vi "ZK组合命令区.vi"(7 "是否启用通讯通知":bool, 8 "error in (no error)":errorcluster, 9 "加标体积":sgl, 10 "组合命令区":T2, 11 "Slave ID":T1) -> (0 "error out":errorcluster)   [LabVIEW 2016, in "质控单元V2.lvlib"]
uses:
  <vilib>/Plasmionique/MB Master/MB_Master/MB_Master.lvclass
  <vilib>/Plasmionique/MB Master/MB Master.lvlib
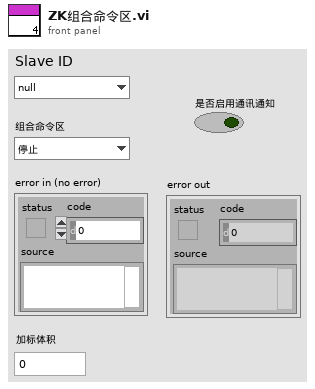
[diagram p1: front panel]
types:
  T1 = typedef "质控单元V2.lvlib/质控slave id.ctl" = enum16{"null", "氨氮", "总磷", "总氮", "CODMn", "CODCr"}
  T2 = typedef "质控单元V2.lvlib/质控组合命令区.ctl" = enum16{"停止", "进水样", "排废液", "进空气（搅拌）", "定量（反转定量）", "加标"}
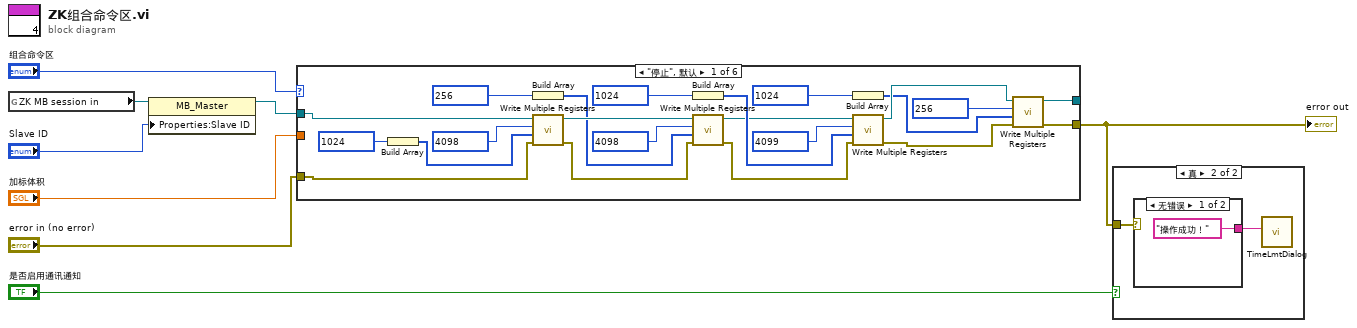
[diagram p0: block diagram]
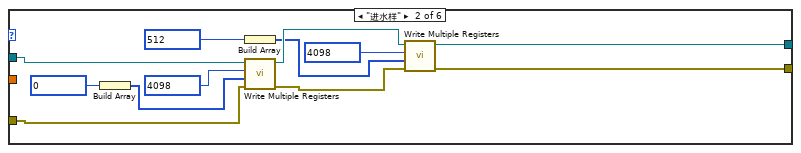
[diagram p2: hidden frame]
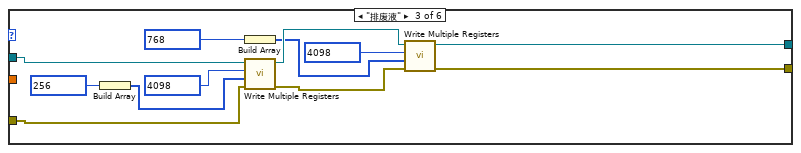
[diagram p3: hidden frame]
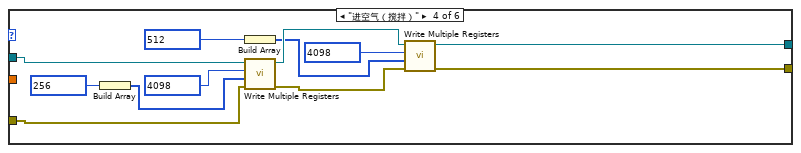
[diagram p4: hidden frame]
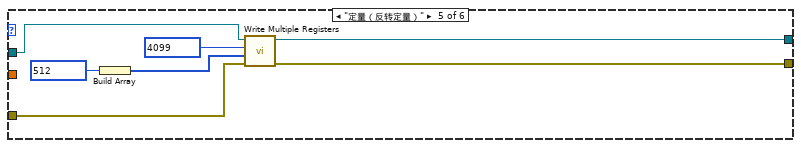
[diagram p5: hidden frame]
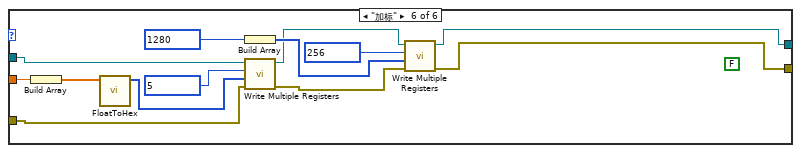
[diagram p6: hidden frame]
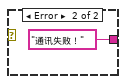
[diagram p8: hidden frame]
diagram:
  n1 = global read "ZK非断电保存全局变量.vi" "ZK MB session in"() -> (w8:refnum<class "MB_Master.lvclass">)
  n2 = property class="MB_Master"(reference=w8, "Properties:Slave ID"="Slave ID") -> (reference out=w5:refnum<class "MB_Master.lvclass">)  [unwired: 1 in, 1 out]
  n3 = case shown="\"停止\", 默认" "组合命令区" {
    tunnel: w5 -> [w29 w41 w53 w65 w72 w78]
    tunnel: "error in (no error)" -> [w27 w40 w52 w64 w71 w76]
    tunnel: [w14 w32 w44 w56 w68 w83] -> _
    tunnel: [w13 w31 w43 w55 w67 w82] -> w1
    tunnel: "加标体积" -> [_ _ _ _ _ w75]
    frame "停止", Default {
      n4 = Build Array(u16 1024 ("starting address")) -> (w9:u16[])
      n5 = Build Array(u16 256 ("starting address")) -> (w22:u16[])
      n6 = call <vilib>:"Write Multiple Registers.vi"("error in (no error)"=w27, "values"=w9, "starting address"=u16 4098, "MB session in"=w29) -> ("error out"=w26:errorcluster, "MB session out"=w25:refnum<class "MB_Master.lvclass">)  [unwired: 6 in]
      n7 = Build Array(u16 1024 ("starting address")) -> (w21:u16[])
      n8 = call <vilib>:"Write Multiple Registers.vi"("error in (no error)"=w26, "values"=w22, "starting address"=u16 4098, "MB session in"=w25) -> ("error out"=w17:errorcluster, "MB session out"=w18:refnum<class "MB_Master.lvclass">)  [unwired: 6 in]
      n9 = Build Array(u16 1024 ("starting address")) -> (w10:u16[])
      n10 = call <vilib>:"Write Multiple Registers.vi"("error in (no error)"=w17, "values"=w21, "starting address"=u16 4099, "MB session in"=w18) -> ("error out"=w15:errorcluster, "MB session out"=w16:refnum<class "MB_Master.lvclass">)  [unwired: 6 in]
      n11 = call <vilib>:"Write Multiple Registers.vi"("error in (no error)"=w15, "values"=w10, "starting address"=u16 256, "MB session in"=w16) -> ("error out"=w13:errorcluster, "MB session out"=w14:refnum<class "MB_Master.lvclass">)  [unwired: 6 in]
    }
    frame "进水样" {
      n12 = Build Array(u16 0 ("starting address")) -> (w38:u16[])
      n13 = Build Array(u16 512 ("starting address")) -> (w34:u16[])
      n14 = call <vilib>:"Write Multiple Registers.vi"("error in (no error)"=w40, "values"=w38, "starting address"=u16 4098, "MB session in"=w41) -> ("error out"=w33:errorcluster, "MB session out"=w37:refnum<class "MB_Master.lvclass">)  [unwired: 6 in]
      n15 = call <vilib>:"Write Multiple Registers.vi"("error in (no error)"=w33, "values"=w34, "starting address"=u16 4098, "MB session in"=w37) -> ("error out"=w31:errorcluster, "MB session out"=w32:refnum<class "MB_Master.lvclass">)  [unwired: 6 in]
    }
    frame "排废液" {
      n16 = Build Array(u16 256 ("starting address")) -> (w50:u16[])
      n17 = Build Array(u16 768 ("starting address")) -> (w46:u16[])
      n18 = call <vilib>:"Write Multiple Registers.vi"("error in (no error)"=w52, "values"=w50, "starting address"=u16 4098, "MB session in"=w53) -> ("error out"=w45:errorcluster, "MB session out"=w49:refnum<class "MB_Master.lvclass">)  [unwired: 6 in]
      n19 = call <vilib>:"Write Multiple Registers.vi"("error in (no error)"=w45, "values"=w46, "starting address"=u16 4098, "MB session in"=w49) -> ("error out"=w43:errorcluster, "MB session out"=w44:refnum<class "MB_Master.lvclass">)  [unwired: 6 in]
    }
    frame "进空气（搅拌）" {
      n20 = Build Array(u16 256 ("starting address")) -> (w62:u16[])
      n21 = Build Array(u16 512 ("starting address")) -> (w58:u16[])
      n22 = call <vilib>:"Write Multiple Registers.vi"("error in (no error)"=w64, "values"=w62, "starting address"=u16 4098, "MB session in"=w65) -> ("error out"=w57:errorcluster, "MB session out"=w61:refnum<class "MB_Master.lvclass">)  [unwired: 6 in]
      n23 = call <vilib>:"Write Multiple Registers.vi"("error in (no error)"=w57, "values"=w58, "starting address"=u16 4098, "MB session in"=w61) -> ("error out"=w55:errorcluster, "MB session out"=w56:refnum<class "MB_Master.lvclass">)  [unwired: 6 in]
    }
    frame "定量（反转定量）" {
      n24 = Build Array(u16 512 ("starting address")) -> (w69:u16[])
      n25 = call <vilib>:"Write Multiple Registers.vi"("error in (no error)"=w71, "values"=w69, "starting address"=u16 4099, "MB session in"=w72) -> ("error out"=w67:errorcluster, "MB session out"=w68:refnum<class "MB_Master.lvclass">)  [unwired: 6 in]
    }
    frame "加标" {
      (unwired) FALSE ("是否启用通讯通知")
      n26 = Build Array(w75) -> (w79:sgl[])
      n27 = call "FloatToHex.vi"("浮点数"=w79) -> ("DCBA整形输出"=w80:u16[])  [unwired: 10 in]
      n28 = Build Array(u16 1280 ("starting address")) -> (w84:u16[])
      n29 = call <vilib>:"Write Multiple Registers.vi"("error in (no error)"=w76, "values"=w80, "starting address"=u16 5, "MB session in"=w78) -> ("error out"=w74:errorcluster, "MB session out"=w77:refnum<class "MB_Master.lvclass">)  [unwired: 6 in]
      n30 = call <vilib>:"Write Multiple Registers.vi"("error in (no error)"=w74, "values"=w84, "starting address"=u16 256, "MB session in"=w77) -> ("error out"=w82:errorcluster, "MB session out"=w83:refnum<class "MB_Master.lvclass">)  [unwired: 6 in]
    }
  }
  "error out" <- w1
  n31 = case shown="真" "是否启用通讯通知" {
    tunnel: w1 -> [_ w88]
    frame False {
    }
    frame True {
      n32 = case shown="无错误" w88 {
        tunnel: ["操作成功！" "通讯失败！"] -> w87
        frame No Error {
        }
        frame Error {
        }
      }
      n33 = call "TimeLmtDialog.vi"("Infoin"=w87) -> ()  [unwired: 11 in]
    }
  }
